vi "Read joystick.vi"(2 "Joystick ID":u32, 5 "error in":errorcluster) -> (14 "XPos":i32, 15 "YPos":i32, 16 "Button 1 pressed":bool, 17 "Button 2 pressed":bool, 19 "error out":errorcluster)   [LabVIEW 2026]
doc: "Sub-VI for operation with a joystick connected to the game port of the host computer. Reads joystick position and button status for a standard 2-button 2-axis joystick. \nInstall joystick driver and calibrate joystick in the Windows control panel before running this VI."
uses:
  winmm.dll
panel:
  out "DLL output":T1
  # "Reads joystick position and button status."
  # "165: bad parameters\n166: request not completed\n167: joystick is unplugged"
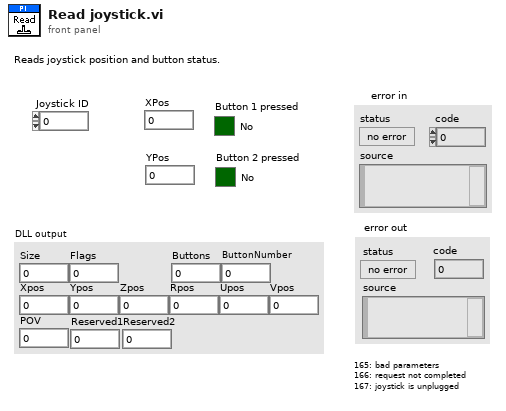
[diagram p1: front panel]
types:
  T1 = cluster{"Size":u32, "Flags":u32, "Xpos":u32, "Ypos":u32, "Zpos":u32, "Rpos":u32, "Upos":u32, "Vpos":u32, "Buttons":u32, "ButtonNumber":u32, "POV":u32, "Reserved1":u32, "Reserved2":u32}
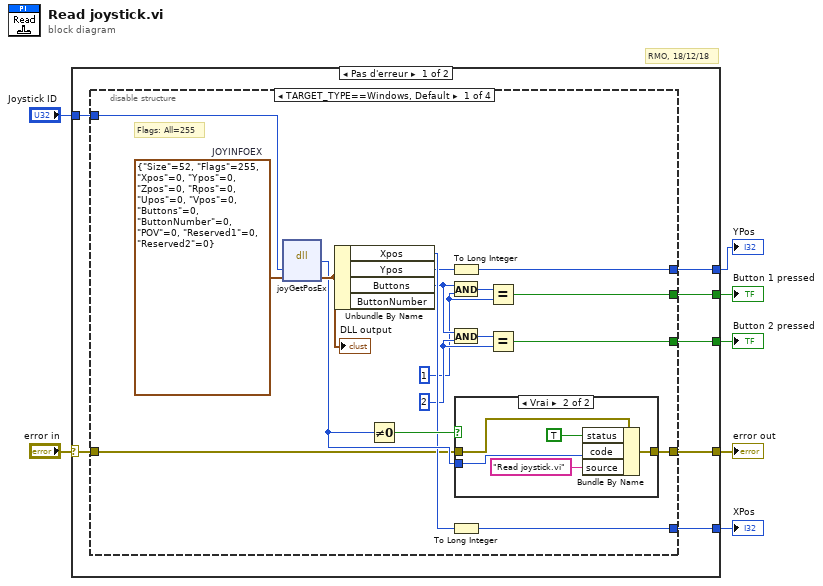
[diagram p0: block diagram]
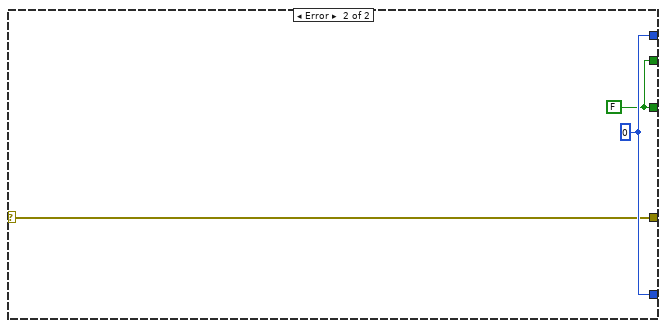
[diagram p6: hidden frame]
diagram:
  # "RMO, 18/12/18"
  n1 = case shown="Pas d'erreur" "error in" {
    selector: "error in" -> [w9 w39]
    tunnel: [w14 w39] -> w7
    tunnel: [w11 w41] -> w6
    tunnel: [w10 w41] -> w5
    tunnel: [w13 w40] -> w4
    tunnel: [w12 w40] -> w3
    tunnel: "Joystick ID" -> [w8 _]
    frame No Error {
      n2 = disable-structure shown="TARGET_TYPE==Windows, Default" {
        disable-tunnel: [w30 _ _ _] -> w14
        disable-tunnel: [w22 _ _ _] -> w13
        disable-tunnel: [w19 _ _ _] -> w12
        disable-tunnel: [w18 _ _ _] -> w11
        disable-tunnel: [w17 _ _ _] -> w10
        disable-tunnel: w9 -> [w16 _ _ _]
        disable-tunnel: w8 -> [w15 _ _ _]
        frame condition #0 (active) {
          w23 = u32 2 ("y")
          w20 = u32 1 ("y")
          w31 = T1 {"Size"=52, "Flags"=255, "Xpos"=0, "Ypos"=0, "Zpos"=0, "Rpos"=0, "Upos"=0, "Vpos"=0, "Buttons"=0, "ButtonNumber"=0, "POV"=0, "Reserved1"=0, "Reserved2"=0}  # JOYINFOEX
          # "Flags: All=255"
          n3 = dll-call lib="winmm.dll" fn="joyGetPosEx"("uJoyID"=w15, "JOYINFOEX"=w31) -> (w28:u32, "JOYINFOEX"=w32:T1)  [unwired: 4 in, 2 out]
          "DLL output" <- w32
          n4 = Unbundle By Name(w32) -> ("Xpos"=w27:u32, "Ypos"=w26:u32, "Buttons"=w25:u32)  [unwired: 1 out]
          n5 = Not Equal To 0?(x=w28) -> (x != 0?=w29:bool)
          n6 = To Long Integer(number=w26) -> (32bit integer=w17:i32)
          n7 = And(x=w25, y=w20) -> (x .and. y?=w21:u32)
          n8 = And(x=w25, y=w23) -> (x .and. y?=w24:u32)
          n9 = To Long Integer(number=w27) -> (32bit integer=w18:i32)
          n10 = case shown="Vrai" w29 {
            tunnel: [w33 w34] -> w30
            tunnel: w16 -> [w33 w38]
            tunnel: w28 -> [_ w36]
            frame False {
            }
            frame True {
              n11 = Bundle By Name(cluster=w38, "status"=TRUE ("Bundle Element"), "code"=w36, "source"="Read joystick.vi" ("Bundle Element")) -> (w34:errorcluster)
            }
          }
          n12 = Equal?(x=w21, y=w20) -> (x = y?=w19:bool)
          n13 = Equal?(x=w24, y=w23) -> (x = y?=w22:bool)
        }
        frame condition #1 {
        }
        frame condition #2 {
        }
        frame condition #3 {
        }
      }
    }
    frame Error {
      w41 = 0 ("Xpos")
      w40 = FALSE
    }
  }
  "error out" <- w7
  "XPos" <- w6
  "YPos" <- w5
  "Button 1 pressed" <- w3
  "Button 2 pressed" <- w4
